vi "FindLongestChain.vi"(0 "object in":refnum<class "StateReverse.lvclass">, 1 "States":T1[](array[typedef]), 2 "State":string, 3 "StateSeqencies":string[](array[string]), 5 "error in (no error)":errorcluster) -> (15 "StateSeqenciesOut":string[](array[string]), 19 "error out":errorcluster)   [LabVIEW 2020, in "StateReverse.lvclass"]
uses:
  <resource>/Framework/Providers/Open_GDS/UML/StateReverse_class/StateReverse.lvclass
  <resource>/Framework/Providers/Open_GDS/UML/ReversedEngineering/ReversedEngineering StateMachineStateInfo.ctl
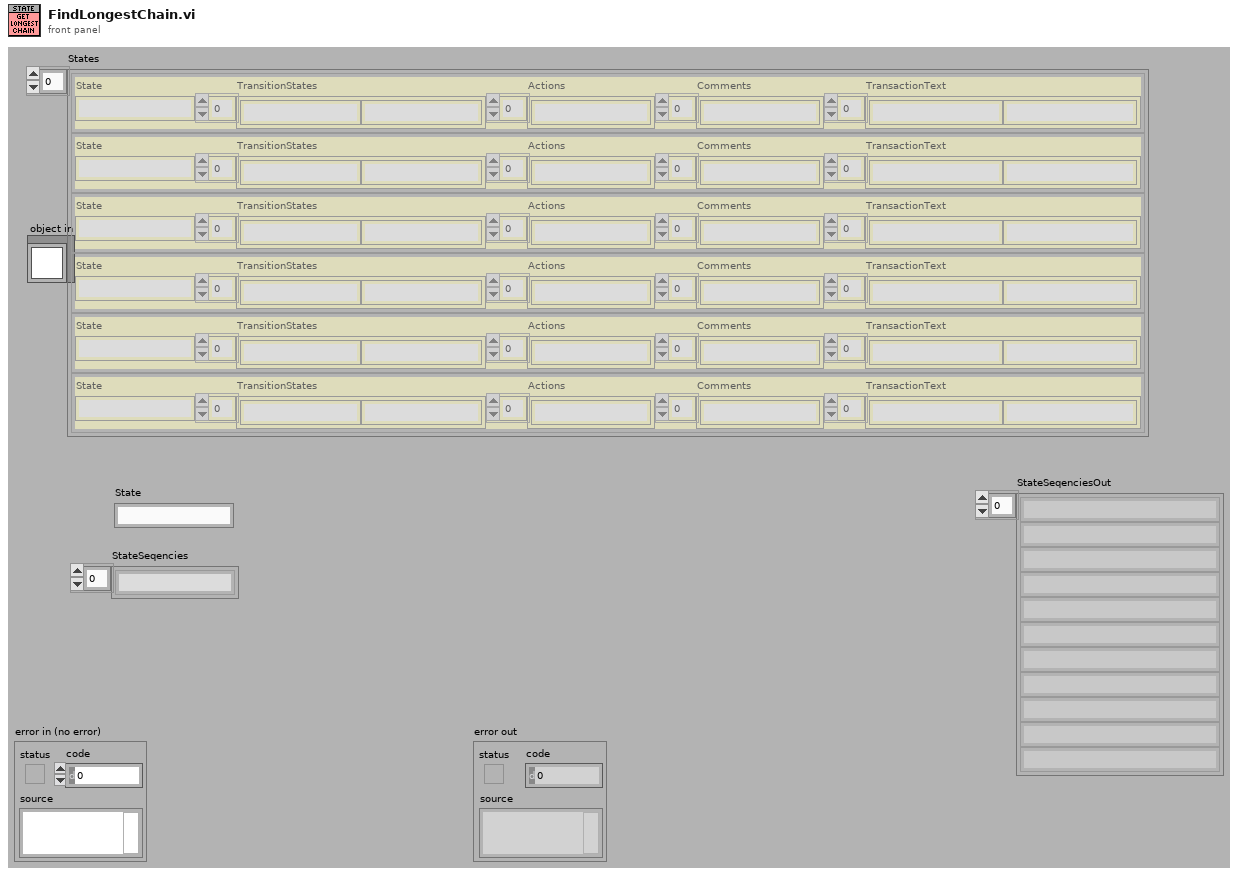
[diagram p1: front panel]
types:
  T1 = typedef "ReversedEngineering StateMachineStateInfo.ctl" = cluster{"State":string, "TransitionStates":string[], "Actions":string[], "Comments":string[], "TransactionText":string[]}
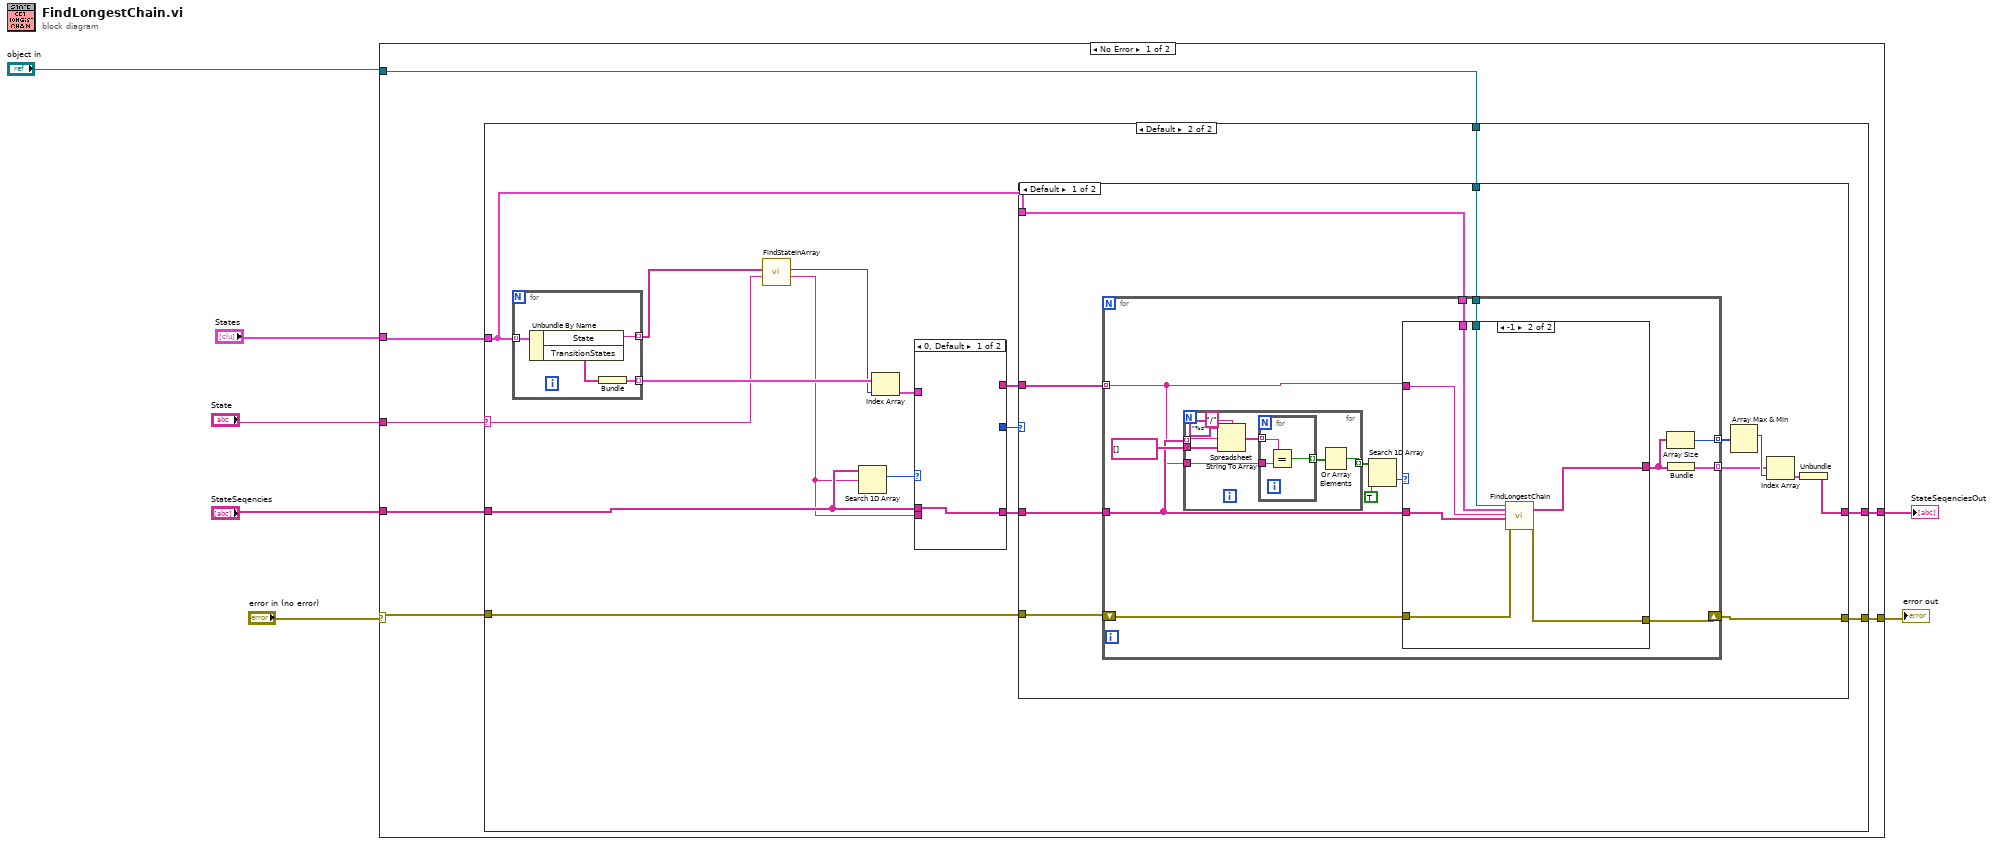
[diagram p0: block diagram]
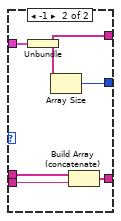
[diagram p3: hidden frame]
diagram:
  n1 = case shown="No Error" "error in (no error)" {
    selector: "error in (no error)" -> [w13 w91]
    tunnel: [w14 w91] -> w6
    tunnel: "object in" -> [w8 _]
    tunnel: "States" -> [w12 _]
    tunnel: "State" -> [w11 _]
    tunnel: "StateSeqencies" -> [w10 w90]
    tunnel: [w9 w90] -> w1
    frame No Error {
      n2 = case shown="Default" w11 {
        selector: w11 -> [_ w22]
        tunnel: [w16 w29] -> w9
        tunnel: w10 -> [w16 w19]
        tunnel: [w15 w27] -> w14
        tunnel: w12 -> [_ w26]
        tunnel: w13 -> [w15 w25]
        tunnel: w8 -> [_ w20]
        frame "" {
        }
        frame Default {
          n3 = for {
            tunnel: w26 -> [w89] mode=indexing
            tunnel: [w88] -> w24 mode=indexing
            tunnel: [w86] -> w32 mode=indexing
            n4 = Unbundle By Name(w89) -> ("State"=w88:string, "TransitionStates"=w87:string[])
            n5 = Bundle("TransitionStates"=w87) -> (w86:cluster{"TransitionStates":string[]})  [unwired: 1 in]
          }
          n6 = call <resource>:"FindStateInArray.vi"("TransactionState"=w22, "AllCaseStates"=w24) -> ("CaseStateOut"=w18:string, "index of element"=w23:i32)  [unwired: 7 in, 1 out]
          n7 = Search 1D Array(1D array=w19, element=w18) -> (index of element=w17:i32)  [unwired: 1 in]
          n8 = Index Array(array=w32, index=w23) -> (element=w30:cluster{"TransitionStates":string[]})
          n9 = case shown="0, Default" w17 {
            tunnel: [_ w39] -> w31
            tunnel: w30 -> [_ w38]
            tunnel: [w33 w37] -> w28
            tunnel: [_ w36] -> w21
            tunnel: w19 -> [w33 w35]
            tunnel: w18 -> [_ w34]
            frame 0, Default {
            }
            frame -1 {
              n10 = Unbundle(w38) -> ("TransitionStates"=w36:string[])
              n11 = Array Size(array=w36) -> (size(s)=w39:i32)
              n12 = Build Array (concatenate)(w35, w34) -> (w37:string[])
            }
          }
          n13 = case shown="Default" w31 {
            tunnel: w21 -> [w47 _]
            tunnel: [w45 w85] -> w29
            tunnel: w28 -> [w46 w85]
            tunnel: w25 -> [w40 w84]
            tunnel: [w41 w84] -> w27
            tunnel: w26 -> [w44 _]
            tunnel: w20 -> [w42 _]
            frame Default {
              n14 = for {
                tunnel: [w60] -> w50 mode=indexing
                tunnel: w47 -> [w52] mode=indexing
                tunnel: w46 -> [w53]
                shift-right: [w62] -> w41
                shift-left: w40 -> [w63]
                tunnel: w44 -> [w61]
                tunnel: [w58] -> w43 mode=indexing
                tunnel: w42 -> [w51]
                n15 = for {
                  tunnel: w53 -> [w71] mode=indexing
                  tunnel: [w64] -> w56 mode=indexing
                  tunnel: string[] [] -> [w69]
                  tunnel: w52 -> [w66]
                  n16 = Spreadsheet String To Array(delimiter (Tab)="/", format string="%s", spreadsheet string=w71, array type (2D Dbl)=w69) -> (array=w67:string[])
                  n17 = for {
                    tunnel: w67 -> [w73] mode=indexing
                    tunnel: w66 -> [w74]
                    tunnel: [w72] -> w65 mode=indexing
                    n18 = Equal?(x=w73, y=w74) -> (x = y?=w72:bool)
                  }
                  n19 = Or Array Elements(Boolean array=w65) -> (logical OR=w64:bool)
                }
                n20 = Search 1D Array(1D array=w56, element=TRUE) -> (index of element=w54:i32)  [unwired: 1 out]
                n21 = case shown="-1" w54 {
                  tunnel: [w76 w80] -> w59
                  tunnel: w63 -> [w75 w79]
                  tunnel: [w75 w78] -> w62
                  tunnel: w53 -> [w76 w81]
                  tunnel: w52 -> [_ w82]
                  tunnel: w61 -> [_ w83]
                  tunnel: w51 -> [_ w77]
                  frame Default {
                    # "This state is already found in the chain,\ndon't use"
                  }
                  frame -1 {
                    n22 = call-dynamic "FindLongestChain.vi"("object in"=w77, "States"=w83, "State"=w82, "StateSeqencies"=w81, "error in (no error)"=w79) -> ("StateSeqenciesOut"=w80:string[], "error out"=w78:errorcluster)  [unwired: 13 in]
                  }
                }
                n23 = Array Size(array=w59) -> (size(s)=w60:i32)
                n24 = Bundle("StateSeqenciesOut"=w59) -> (w58:cluster{"StateSeqenciesOut":string[]})  [unwired: 1 in]
              }
              n25 = Array Max & Min(array=w50) -> (max index (indices)=w49:i32)  [unwired: 3 out]
              n26 = Index Array(array=w43, index=w49) -> (element=w48:cluster{"StateSeqenciesOut":string[]})
              n27 = Unbundle(w48) -> ("StateSeqenciesOut"=w45:string[])
            }
            frame 0 {
            }
          }
        }
      }
    }
    frame Error {
    }
  }
  "error out" <- w6
  "StateSeqenciesOut" <- w1
